vi "Recording Path.vi"(8 "error in (no error)":errorcluster, 11 "AcquistionObject in":refnum<class "AcquistionObject.lvclass">) -> (0 "error out":errorcluster, 2 "FilePath":path, 3 "AcquistionObject out":refnum<class "AcquistionObject.lvclass">)   [LabVIEW 2012, in "AcquisitionCoreLibrary.lvlib" / "AcquistionObject.lvclass"]
uses:
  AcquistionObject.lvclass
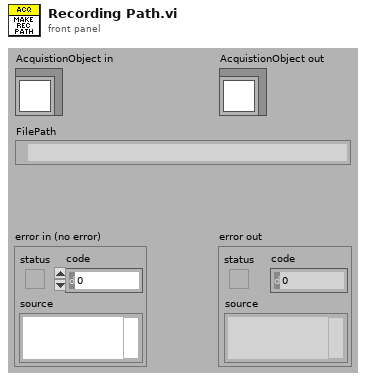
[diagram p1: front panel]
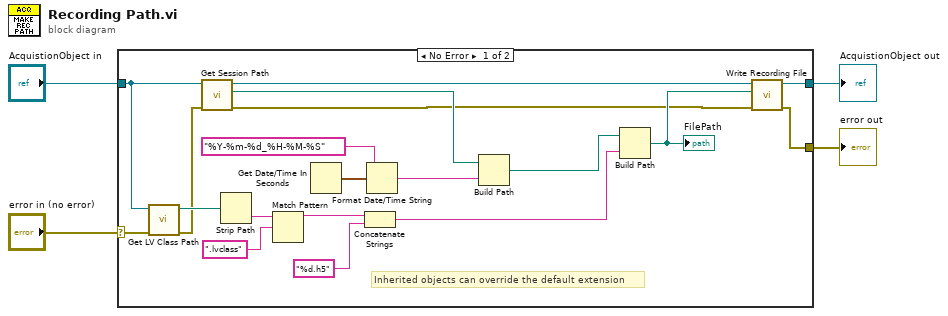
[diagram p0: block diagram]
diagram:
  n1 = case shown="No Error" "error in (no error)" {
    selector: "error in (no error)" -> [w13 w25]
    tunnel: [w15 w25] -> w3
    tunnel: [w17 w24] -> w1
    tunnel: "AcquistionObject in" -> [w12 w24]
    frame No Error {
      # "Inherited objects can override the default extension"
      n2 = call <vilib>:"Get LV Class Path.vi"("error in (no error)"=w13, "object"=w12) -> ("error out"=w14:errorcluster, "class path"=w21:path)  [unwired: 8 in]
      n3 = call-dynamic "Get Session Path.vi"("error in (no error)"=w14, "AcquistionObject in"=w12) -> ("error out"=w5:errorcluster, "Path"=w18:path, "AcquistionObject out"=w11:refnum<class "AcquistionObject.lvclass">)  [unwired: 7 in]
      n4 = Strip Path(path=w21) -> (name=w9:string)  [unwired: 1 out]
      n5 = Match Pattern(string=w9, regular expression=".lvclass") -> (before substring=w7:string)  [unwired: 1 in, 3 out]
      n6 = Get Date/Time In Seconds() -> (seconds since 1Jan1904=w22:timestamp)
      n7 = Concatenate Strings(w7, "%d.h5" ("string")) -> (w19:string)
      n8 = Format Date/Time String(time format string (%c)="%Y-%m-%d_%H-%M-%S", seconds (now)=w22) -> (date/time string=w20:string)  [unwired: 1 out]
      n9 = Build Path(base path=w18, name or relative path=w20) -> (appended path=w6:path)
      n10 = Build Path(base path=w6, name or relative path=w19) -> (appended path=w16:path)
      "FilePath" <- w16
      n11 = call-dynamic "Write Recording File.vi"("error in (no error)"=w5, "Recording File"=w16, "AcquistionObject in"=w11) -> ("error out"=w15:errorcluster, "AcquistionObject out"=w17:refnum<class "AcquistionObject.lvclass">)  [unwired: 7 in]
    }
    frame Error {
    }
  }
  "error out" <- w3
  "AcquistionObject out" <- w1
